vi "Get Pre Amp Gain Text.vi"(8 "error in (no error)":errorcluster, 9 "length":i32, 10 "name":string, 11 "index":i32) -> (0 "error out":errorcluster, 2 "name out":string, 3 "function return":u32)   [LabVIEW 2014, in "atmcd32d.lvlib"]
doc: "unsigned int WINAPI GetPreAmpGainText(int index, char * name, int length);"
uses:
  atmcd32d.lvlib
  atmcd32d.dll
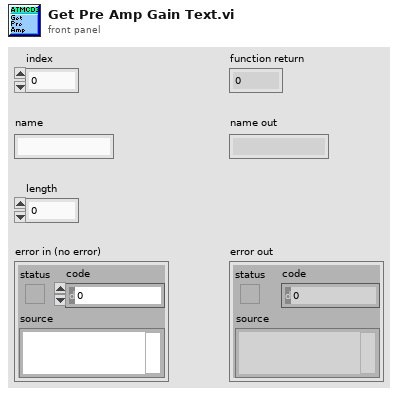
[diagram p1: front panel]
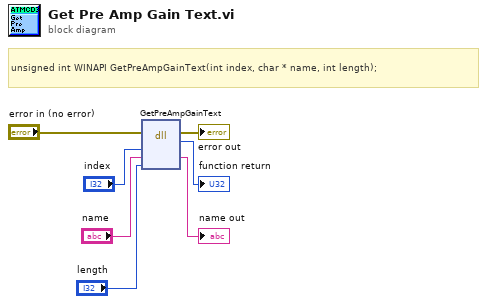
[diagram p0: block diagram]
diagram:
  # "unsigned int WINAPI GetPreAmpGainText(int index, char * name, int length);"
  n1 = dll-call lib="C:/Users/Bakir/Documents/Lambda2-Testing/lib/Andorlib/atmcd32d.*" fn="GetPreAmpGainText"(error in="error in (no error)", "index"="index", "name"="name", "length"="length") -> (error out=→"error out":errorcluster, →"function return":u32, "name"=→"name out":string)  [unwired: 4 in, 1 out]
